vi "Write Character Set.vi"(8 "error in (no error)":errorcluster, 10 "Character Set":T1, 11 "ZXing Options in":refnum<class "ZXing Options.lvclass">) -> (0 "error out":errorcluster, 3 "ZXing Options out":refnum<class "ZXing Options.lvclass">)   [LabVIEW 2020, in "feature_detection.lvlib" / "ZXing Options.lvclass"]
uses:
  ZXing Options.lvclass
  ZXing Options.lvclass/ZXing Options.ctl
  Field.ctl
  Character Set.ctl
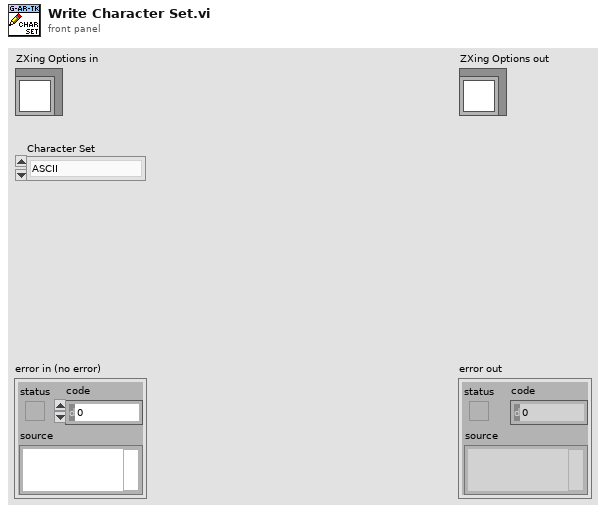
[diagram p1: front panel]
types:
  T1 = typedef "feature_detection.lvlib/ZXing Options.lvclass/Character Set.ctl" = enum8{"ASCII", "ISO8859_1", "ISO8859_2", "ISO8859_3", "ISO8859_4", "ISO8859_5", "ISO8859_6", "ISO8859_7", "ISO8859_8", "ISO8859_9", "ISO8859_10", "ISO8859_11", "ISO8859_13", "ISO8859_14", "ISO8859_15", "ISO8859_16", "Cp437", "Cp1250", "Cp1251", "Cp1252", "Cp1256", "Shift_JIS", "Big5", "GB2312", "GB18030", "EUC_JP", "EUC_KR", "UTF16BE", "UTF8", "UTF16LE", "UTF32BE", "UTF32LE", "BINARY"}
  T2 = typedef "feature_detection.lvlib/ZXing Options.lvclass/Field.ctl" = enum8{"Try Harder", "Try Rotate", "Try Invert", "Try Downscale", "Is Pure", "Try Code 39 Ext Mode", "Return Errors", "Downscale Factor", "Min Line Count", "Max Number of Symbols", "Binarizer", "EAN Add On Symbol", "Text Mode", "Character Set", "Downscale Threshold"}
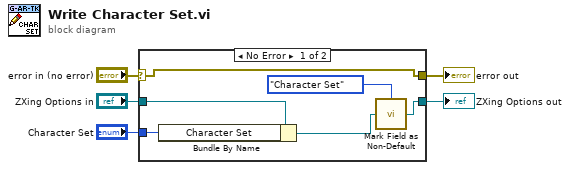
[diagram p0: block diagram]
diagram:
  n1 = case shown="No Error" "error in (no error)" {
    selector: "error in (no error)" -> [w11 w12]
    tunnel: [w11 w12] -> w4
    tunnel: [w7 w13] -> w2
    tunnel: "ZXing Options in" -> [w10 w13]
    tunnel: "Character Set" -> [w8 _]
    frame No Error {
      n2 = Bundle By Name(cluster=w10, "Character Set"=w8) -> (w9:refnum<class "ZXing Options.lvclass">)
      n3 = call "Mark Field as Non-Default.vi"("ZXing Options in"=w9, "Field"=Field."Character Set") -> ("ZXing Options out"=w7:refnum<class "ZXing Options.lvclass">)
    }
    frame Error {
    }
  }
  "error out" <- w4
  "ZXing Options out" <- w2
